vi "GetTextReference.vi"(8 "error in":errorcluster, 11 "Decoration in":refnum<class "Decoration.lvclass">) -> (0 "error out":errorcluster, 1 "Text reference":refnum<vi>, 3 "Decoration out":refnum<class "Decoration.lvclass">)   [LabVIEW 2014, in "Raspberry Pi Compatible Compiler for LabVIEW.lvlib" / "Text.lvclass"]
uses:
  Text.lvclass
  Decoration/Decoration.lvclass
  Generic/Generic.lvclass
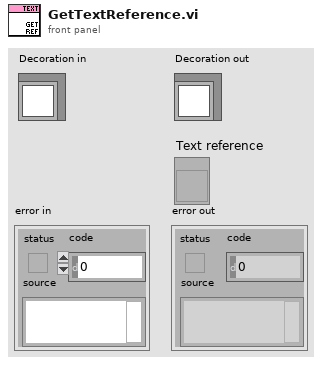
[diagram p1: front panel]
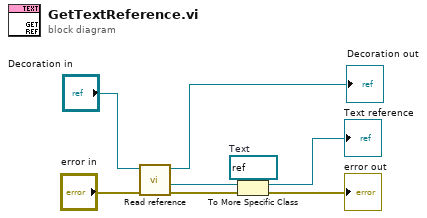
[diagram p0: block diagram]
diagram:
  w8 = refnum<vi> refnum  # Text
  n1 = call "Read reference.vi"("error in"="error in", "GObject in"="Decoration in") -> ("error out"=w3:errorcluster, "reference"=w2:refnum<vi>, "GObject out"=→"Decoration out":refnum<class "Decoration.lvclass">)  [unwired: 5 in]
  n2 = To More Specific Class(target class=w8, reference=w2, error in=w3) -> (specific class reference=→"Text reference":refnum<vi>, error out=→"error out":errorcluster)
